vi "SCLN_Authenticate.vi"(2 "TCP IN":refnum<k5>, 3 "Server Number":i32, 4 "Computer Name":string) -> (0 "TCP OUT":refnum<k5>, 1 "Authentic":bool)   [LabVIEW 2015]
uses:
  SCLN_RW_Select.ctl
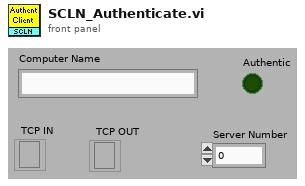
[diagram p1: front panel]
types:
  T1 = typedef "SCLN_RW_Select.ctl" = enum16{"Read", "Write"}
  T2 = typedef "SCLN_InfoClusterConfig.ctl" = cluster{"Section Name":string, "IP_Server":string, "IP_Client":string, "IP_Port":string}
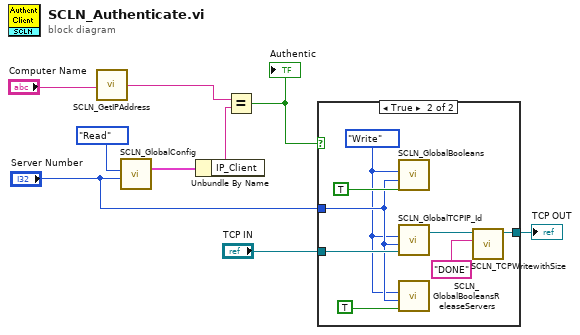
[diagram p0: block diagram]
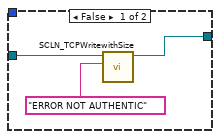
[diagram p2: hidden frame]
diagram:
  n1 = call "SCLN_GetIPAddress.vi"("Computer Name"="Computer Name") -> ("IP Address"=w5:string)
  n2 = call "SCLN_GlobalConfig.vi"("Element"="Server Number", "Operation"=SCLN_RW_Select."Read" ("GBL_RW")) -> ("Read Value"=w7:T2)  [unwired: 2 in, 1 out]
  n3 = Unbundle By Name(w7) -> ("IP_Client"=w6:string)
  n4 = Equal?(x=w5, y=w6) -> (x = y?=w4:bool)
  "Authentic" <- w4
  n5 = case shown="True" w4 {
    tunnel: "Server Number" -> [_ w15]
    tunnel: "TCP IN" -> [w12 w19]
    tunnel: [w11 w16] -> w1
    frame False {
      n6 = call "SCLN_TCPWritewithSize.vi"("data in"="ERROR NOT AUTHENTIC", "connection ID"=w12) -> ("connection ID out"=w11:refnum<k5>)  [unwired: 7 in, 2 out]
    }
    frame True {
      w14 = SCLN_RW_Select."Write" ("GBL_RW")
      n7 = call "SCLN_GlobalBooleans.vi"("Write Value"=TRUE, "Element"=w15, "Operation"=w14) -> ()  [unwired: 1 in, 2 out]
      n8 = call "SCLN_GlobalTCPIP_Id.vi"("TCPIP_Id Write"=w19, "Element"=w15, "Operation"=w14) -> ("TCPIP_Id Read"=w17:refnum<k5>)  [unwired: 1 in, 1 out]
      n9 = call "SCLN_GlobalBooleansReleaseServers.vi"("Write Value"=TRUE, "Element"=w15, "Operation"=w14) -> ()  [unwired: 1 in, 2 out]
      n10 = call "SCLN_TCPWritewithSize.vi"("data in"="DONE", "connection ID"=w17) -> ("connection ID out"=w16:refnum<k5>)  [unwired: 7 in, 2 out]
    }
  }
  "TCP OUT" <- w1
